vi "6.2.2.-Lógica Difusa SIMO Carrito - Giro.vi"() -> ()   [LabVIEW 2020]
uses:
  <vilib>/addons/Fuzzy Logic/FL Fuzzy Controller (SIMO).vi
  <vilib>/addons/Fuzzy Logic/NI_Fuzzy_Logic_API.lvlib
panel:
  out "Plano de trabajo":picture
  out "Meter":dbl(knob) scale=-25.0..25.0
  out "Tank":dbl(slide) scale=0.0..10.0
  in  "Reset":bool
  out "Motor Izquierda":dbl(slide) scale=-100.0..100.0
  out "Motor Derecha":dbl(slide) scale=-100.0..100.0
  in  "stop":bool
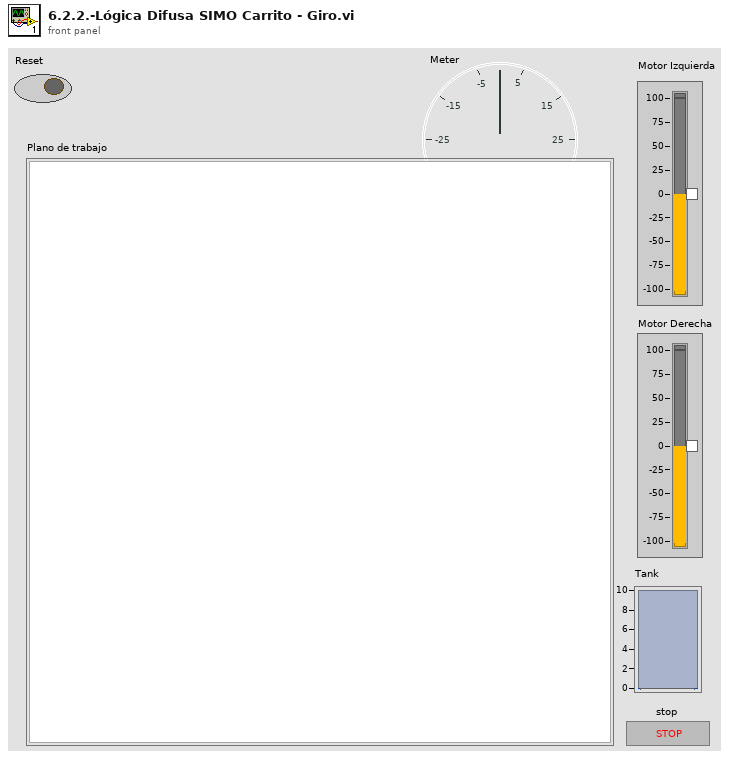
[diagram p1: front panel]
types:
  T1 = typedef "NI_Fuzzy_Logic_API.lvlib/FL System.ctl" = cluster{"input variables":T2[], "output variables":T2[], "rules":T5[], "defuzzification method":T11, "description":string, "user MF interpolating polynomials":T12[]}
  T2 = typedef "NI_Fuzzy_Logic_API.lvlib/FL Variable.ctl" = cluster{"name":string, "range":dbl[], "MFs":T3[]}
  T3 = typedef "NI_Fuzzy_Logic_API.lvlib/FL Membership Function.ctl" = cluster{"name":string, "shape":T4, "points":dbl[], "color":u32, "user-defined shape index":i32}
  T4 = typedef "NI_Fuzzy_Logic_API.lvlib/FL Membership Function Shape.ctl" = u16
  T5 = typedef "NI_Fuzzy_Logic_API.lvlib/FL Rule.ctl" = cluster{"antecedents":T6[], "antecedent connective":T8, "consequents":T9[], "consequent implication":T10, "degree of support":dbl}
  T6 = typedef "NI_Fuzzy_Logic_API.lvlib/FL Antecedent.ctl" = cluster{"Var Index":i32, "MF Index":i32, "Cond":T7}
  T7 = typedef "NI_Fuzzy_Logic_API.lvlib/FL Modifier.ctl" = u16
  T8 = typedef "NI_Fuzzy_Logic_API.lvlib/FL Antecedent Connective.ctl" = u16
  T9 = typedef "NI_Fuzzy_Logic_API.lvlib/FL Consequent.ctl" = cluster{"Var Index":i32, "MF Index":i32, "Cond":T7}
  T10 = typedef "NI_Fuzzy_Logic_API.lvlib/FL Consequent Implication.ctl" = u16
  T11 = typedef "NI_Fuzzy_Logic_API.lvlib/FL Defuzzification.ctl" = u16
  T12 = typedef "NI_Fuzzy_Logic_API.lvlib/FL Interpolating polynomials.ctl" = cluster{"X":dbl[], "Y":dbl[], "Y(x) coeff":dbl[][], "X(y) coeff":dbl[][], "Area(y) coeff":dbl[][], "coa_x(y) coeff":dbl[][]}
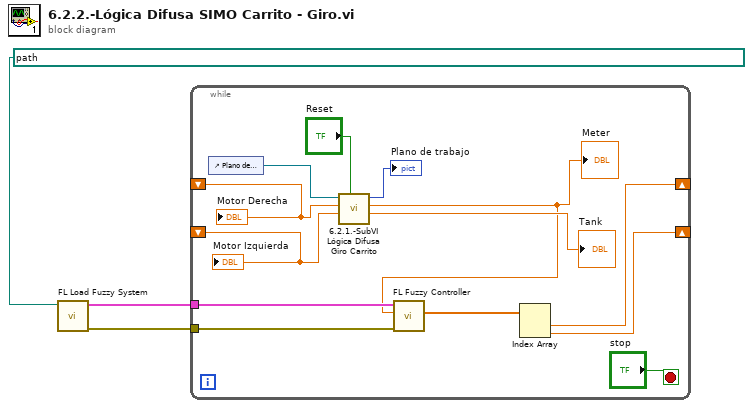
[diagram p0: block diagram]
diagram:
  n1 = call <vilib>:"FL Load Fuzzy System.vi"("file path"=path "C:/Users/diego/OneDrive/Documents/Aprendiendo/LabVIEW/1.-Sistemas de Visión Artificial/6.2.0.-Modelo Lógica Difusa Giro Carrito.fs") -> ("error out"=w1:errorcluster, "fuzzy system out"=w2:T1)  [unwired: 9 in]
  n2 = while {
    tunnel: w2 -> [w12]
    tunnel: w1 -> [w11]
    shift-right: [w7] -> _
    shift-left: _ -> [w5]
    shift-right: [w6] -> _
    shift-left: _ -> [w4]
    stop <- "stop" stop-if-true
    n3 = control-ref of="Plano de trabajo"() -> (w9:refnum<vi>)
    n4 = call "6.2.1.-SubVI Lógica Difusa Giro Carrito.vi"("Reset"="Reset", "Motor Izquierda"=w4, "Motor Derecha"=w5, "Ref Plano"=w9) -> ("Distancia"=→"Tank":dbl, "Angulo"=w10:dbl, "Plano de trabajo"=→"Plano de trabajo":picture)  [unwired: 3 in, 2 out]
    "Meter" <- w10
    n5 = call-poly <vilib>:"FL Fuzzy Controller.vi"("error in (no error)"=w11, "input value"=w10, "fuzzy system in"=w12) -> ("output values"=w8:dbl[])  [unwired: 4 in, 4 out]
    n6 = Index Array "Index Array"(array=w8) -> (element #1=w7:dbl, element #2=w6:dbl)  [unwired: 2 in]
    "Motor Derecha" <- w5
    "Motor Izquierda" <- w4
  }
